vi "terminate.vi"(8 "error in (no error)":errorcluster, 11 "GenericPlugin in":refnum<class "TrajectoryAK101022Resonance.lvclass">) -> (0 "error out":errorcluster, 3 "GenericPlugin out":refnum<class "TrajectoryAK101022Resonance.lvclass">)   [LabVIEW 2010, in "TrajectoryAK101022Resonance.lvclass"]
doc: "The dynamic dispatch version of this VI terminates the plug-in object by releasing all of its resources."
uses:
  TrajectoryAK101022Resonance.lvclass
  TrajectoryAK101022Resonance.lvclass/TrajectoryAK101022Resonance.ctl
  TrajectoryMG100122GenericFPGA/TrajectoryMG100122GenericFPGA/TrajectoryMG100122GenericFPGA.lvclass
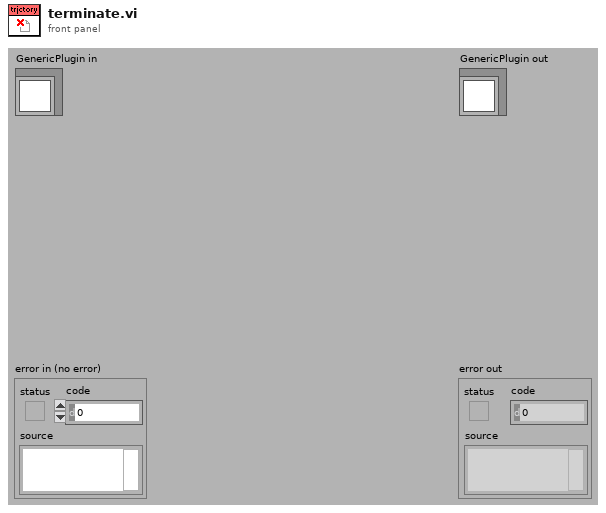
[diagram p1: front panel]
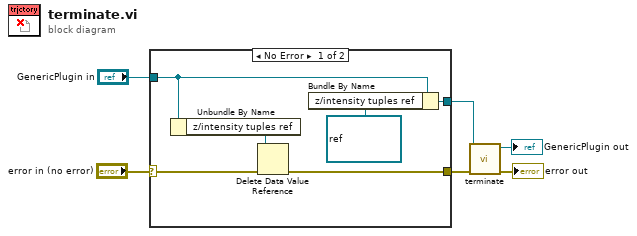
[diagram p0: block diagram]
diagram:
  n1 = case shown="No Error" "error in (no error)" {
    selector: "error in (no error)" -> [w11 w14]
    tunnel: [w12 w14] -> w4
    tunnel: "GenericPlugin in" -> [w9 w13]
    tunnel: [w8 w13] -> w1
    frame No Error {
      n2 = Unbundle By Name(w9) -> ("z/intensity tuples ref"=w10:refnum<data-value>)
      n3 = Delete Data Value Reference(data value reference=w10, error in=w11) -> (error out=w12:errorcluster)  [unwired: 1 out]
      n4 = Bundle By Name(cluster=w9, "z/intensity tuples ref"=refnum<data-value> refnum) -> (w8:refnum<class "TrajectoryAK101022Resonance.lvclass">)
    }
    frame Error {
    }
  }
  n5 = call-parent "terminate.vi"("error in (no error)"=w4, "GenericPlugin in"=w1) -> ("error out"=→"error out":errorcluster, "GenericPlugin out"=→"GenericPlugin out":refnum<class "TrajectoryAK101022Resonance.lvclass">)  [unwired: 8 in]
